vi "Read.vi"(11 "ChannelValue in":refnum<class "StringChannelValue.lvclass">) -> (2 "Channel":refnum<class "Channel STR.lvclass">)   [LabVIEW 2020, in "Vecto.lvlib" / "StringChannelValue.lvclass"]
uses:
  StringChannelValue.lvclass
  Channel STR/Channel STR.lvclass
  StringChannelValue.lvclass/StringChannelValue.ctl
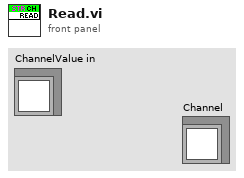
[diagram p1: front panel]
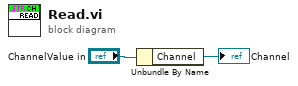
[diagram p0: block diagram]
diagram:
  n1 = Unbundle By Name("ChannelValue in") -> ("Channel"=→"Channel":refnum<class "Channel STR.lvclass">)
